vi "Bounce Window_User Accounts_SubVI_Time.vi"(11 "期限：":T1=enum."一天") -> (2 "期限":string, 3 "目前時間":string)   [LabVIEW 2015]
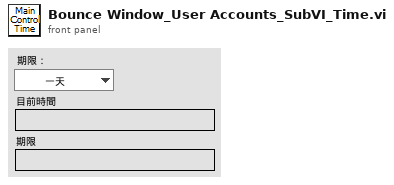
[diagram p1: front panel]
types:
  T1 = typedef "Control_User account_Date.ctl" = enum16{"零天", "一天", "七天", "一個月", "一年", "三年"}
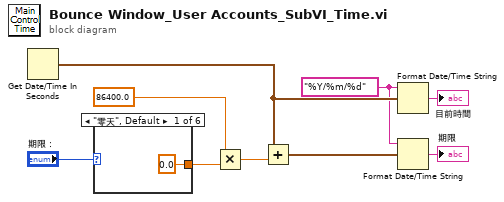
[diagram p0: block diagram]
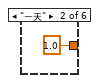
[diagram p2: hidden frame]
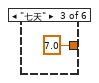
[diagram p3: hidden frame]
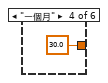
[diagram p4: hidden frame]
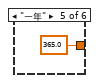
[diagram p5: hidden frame]
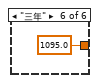
[diagram p6: hidden frame]
diagram:
  w1 = "%Y/%m/%d" ("time format string (%c)")
  n1 = Get Date/Time In Seconds() -> (seconds since 1Jan1904=w2:timestamp)
  n2 = case shown="\"零天\", Default" "期限：" {
    tunnel: [0.0 ("y") 1.0 ("y") 7.0 ("y") 30.0 ("y") 365.0 ("y") 1095.0 ("y")] -> w6
    frame "零天", Default {
    }
    frame "一天" {
    }
    frame "七天" {
    }
    frame "一個月" {
    }
    frame "一年" {
    }
    frame "三年" {
    }
  }
  n3 = Multiply(x=86400.0 ("y"), y=w6) -> (x*y=w5:dbl)
  n4 = Add(x=w2, y=w5) -> (x+y=w3:timestamp)
  n5 = Format Date/Time String(time format string (%c)=w1, seconds (now)=w2) -> (date/time string=→"目前時間":string)  [unwired: 1 in]
  n6 = Format Date/Time String(time format string (%c)=w1, seconds (now)=w3) -> (date/time string=→"期限":string)  [unwired: 1 in]
